vi "WaveSave.vi"() -> ()   [LabVIEW 2014]
uses:
  <vilib>/Analysis/NI_AALBase.lvlib
panel:
  out "rate":u32
  in  "Sound Format":T1={"sound quality"=enum."stereo", "rate"=44100} {"rate" min=4000 step=1000}
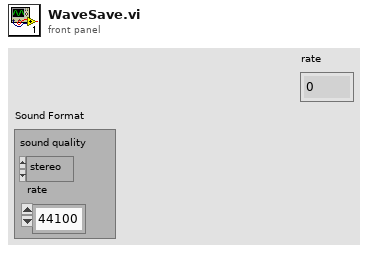
[diagram p1: front panel]
types:
  T1 = cluster{"sound quality":enum16{"mono", "stereo"}, "rate":u32}
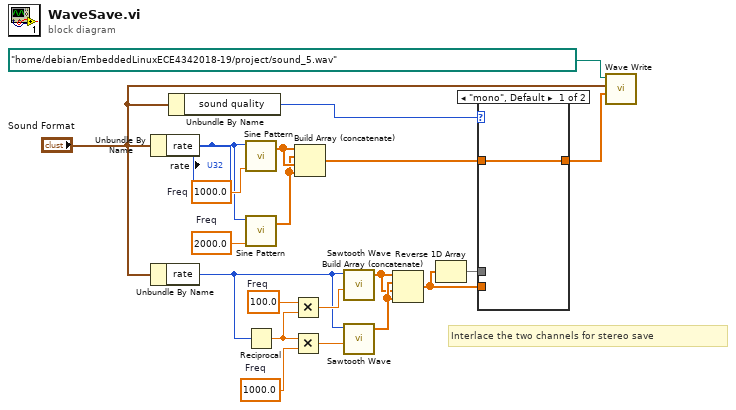
[diagram p0: block diagram]
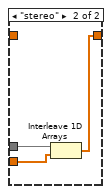
[diagram p2: hidden frame]
diagram:
  w4 = 1000.0  # Freq
  w8 = 100.0  # Freq
  w19 = 2000.0  # Freq
  w20 = 1000.0  # Freq
  # "Interlace the two channels for stereo save"
  n1 = Unbundle By Name("Sound Format") -> ("rate"=w14:u32)
  "rate" <- w14
  n2 = Unbundle By Name("Sound Format") -> ("rate"=w6:u32)
  n3 = Unbundle By Name("Sound Format") -> ("sound quality"=w13:enum16{"mono", "stereo"})
  n4 = call <vilib>:"Sine Pattern.vi"("cycles"=w20, "samples"=w14) -> ("Sinusoidal Pattern"=w18:dbl[])  [unwired: 2 in, 1 out]
  n5 = call <vilib>:"Sine Pattern.vi"("cycles"=w19, "samples"=w14) -> ("Sinusoidal Pattern"=w17:dbl[])  [unwired: 2 in, 1 out]
  n6 = Reciprocal(x=w6) -> (1/x=w5:dbl)
  n7 = Multiply(x=w8, y=w5) -> (x*y=w7:dbl)
  n8 = Multiply(x=w5, y=w4) -> (x*y=w3:dbl)
  n9 = Build Array (concatenate)(w18, w17, w18, w17) -> (w16:dbl[])
  n10 = call <vilib>:"Sawtooth Wave.vi"("samples"=w6, "frequency"=w7) -> ("sawtooth wave"=w10:dbl[])  [unwired: 3 in, 2 out]
  n11 = call <vilib>:"Sawtooth Wave.vi"("samples"=w6, "frequency"=w3) -> ("sawtooth wave"=w11:dbl[])  [unwired: 3 in, 2 out]
  n12 = Build Array (concatenate)(w10, w11, w10, w11) -> (w2:dbl[])
  n13 = Reverse 1D Array(array=w2) -> (reversed array=w1:dbl[])
  n14 = case shown="\"mono\", Default" w13 {
    tunnel: w16 -> [w21 _]
    tunnel: [w21 w24] -> w15
    tunnel: w2 -> [_ w23]
    tunnel: w1 -> [_ w22]
    frame "mono", Default {
    }
    frame "stereo" {
      n15 = Interleave 1D Arrays(w22, w23) -> (w24:dbl[])
    }
  }
  n16 = call "Wave Write.vi"("Audio Input (+/- 1)"=w15, "Sound Format"="Sound Format", "File Path"=path "/home/debian/EmbeddedLinuxECE4342018-19/project/sound_5.wav" ("file path (use dialog)")) -> ()  [unwired: 8 in, 1 out]
